vi "Set_Power_Ref(SA).vi"(0 "Spectrum Analyzer":refnum<visa-resource-name>="TCPIP0::K-N90X0A-00005.local::inst0::INSTR", 1 "P_REF":dbl=41.5, 3 "SG_Offset":dbl=26.9, 5 "SigGen1":refnum<visa-resource-name>="GPIB0::18::INSTR", 9 "RF Freq (MHz)":dbl=1840.0, 11 "error in (no error)":errorcluster {"code" format="%.0x"}, 12 "Start Power (dBm)":dbl=15.0, 13 "accuracy +/-":sgl(ring)=0.2 items=["0.1"=0.1, "0.2"=0.2, "0.3"=0.3, "0.4"=0.4, "0.5"=0.5, "1"=1, "2"=2], 14 "Pin MAX":dbl=25.0) -> (4 "Pin (RF1) str":string="51.03", 6 "Pin (RF)":dbl=51.03, 10 "Elasped time(s)":dbl=8.86637079998036, 15 "error out":errorcluster {"code" format="%.0x"})   [LabVIEW 2018]
panel:
  out "SG_Delay(s)":sgl=2.0
  out "x+y":dbl
  in  "Set to Cont Sweep at End":bool
  in  "SA Timeout":u32=3000
  out "End Time":dbl=154195.45798069998 format="%_19f"
  out "Start Time":dbl=154186.5916099 format="%_19f"
  out "ONE_SHOT_Pin":dbl=24.728961346
  out "One Shot >?":bool=TRUE
  out "ONE_SHOT_Pout":dbl=41.992924491
  out "In Range?":bool=TRUE
  out "INIT_DELTA":dbl=9.728961345999998
  out "INIT_GAIN":dbl=16.771038654
  out "INIT_Pout":dbl=31.771038654
  out "P_REF_H":dbl=41.70000000298023
  out "P_REF_L":dbl=41.399999998509884
  out "Power (dBm)":dbl=41.430916708
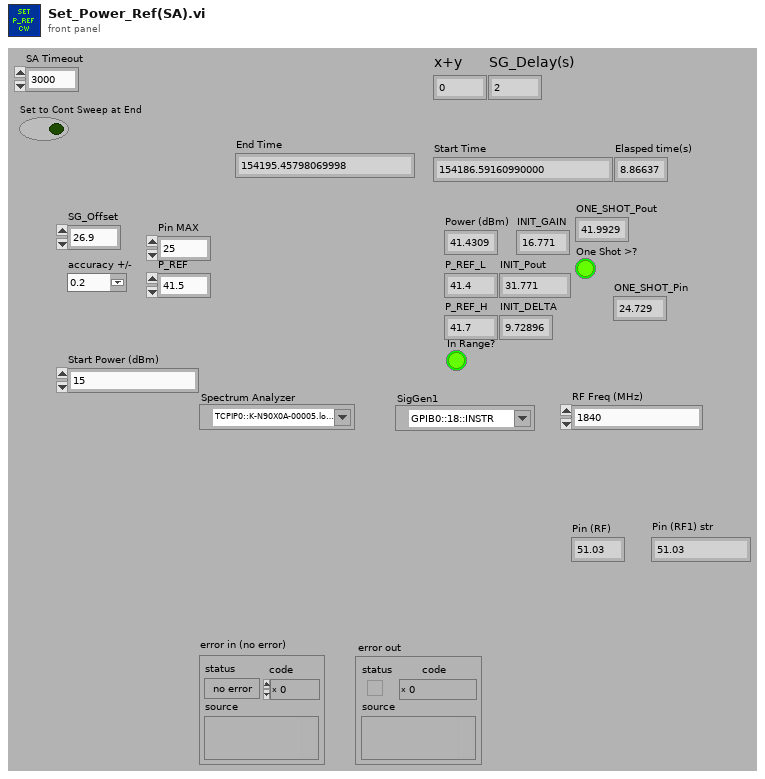
[diagram p1: front panel]
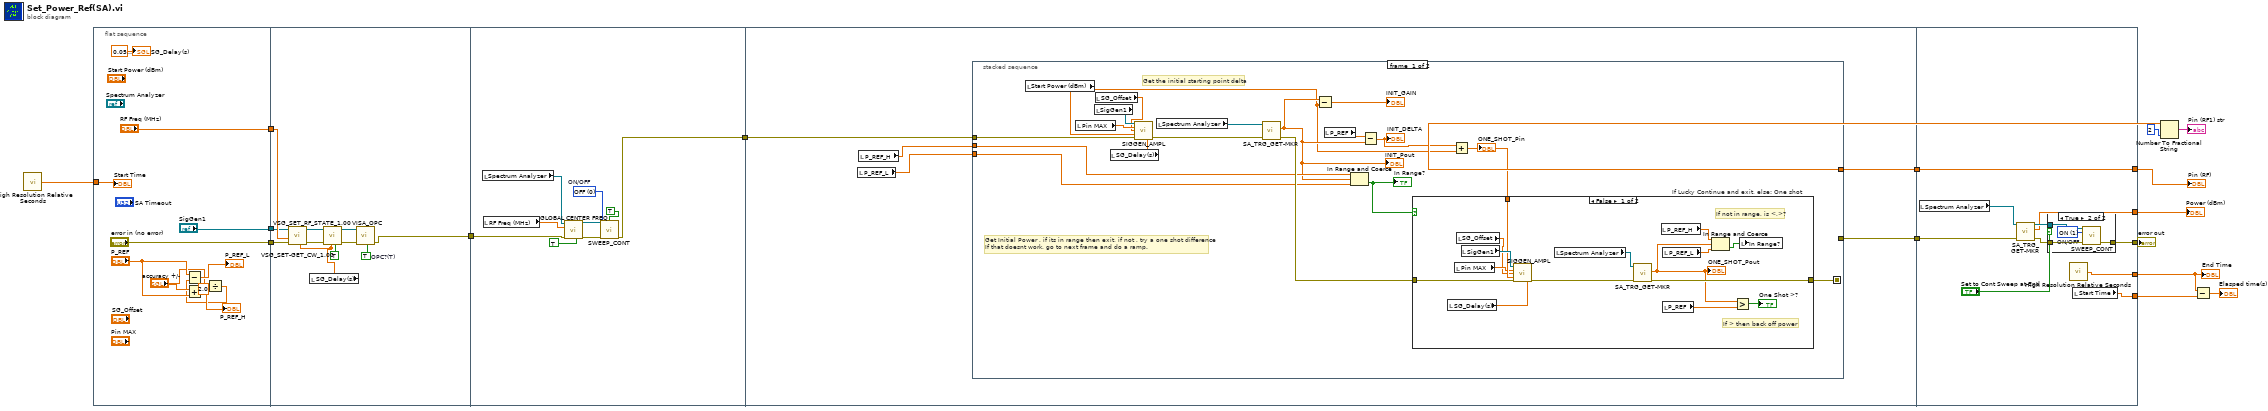
[diagram p0: block diagram]
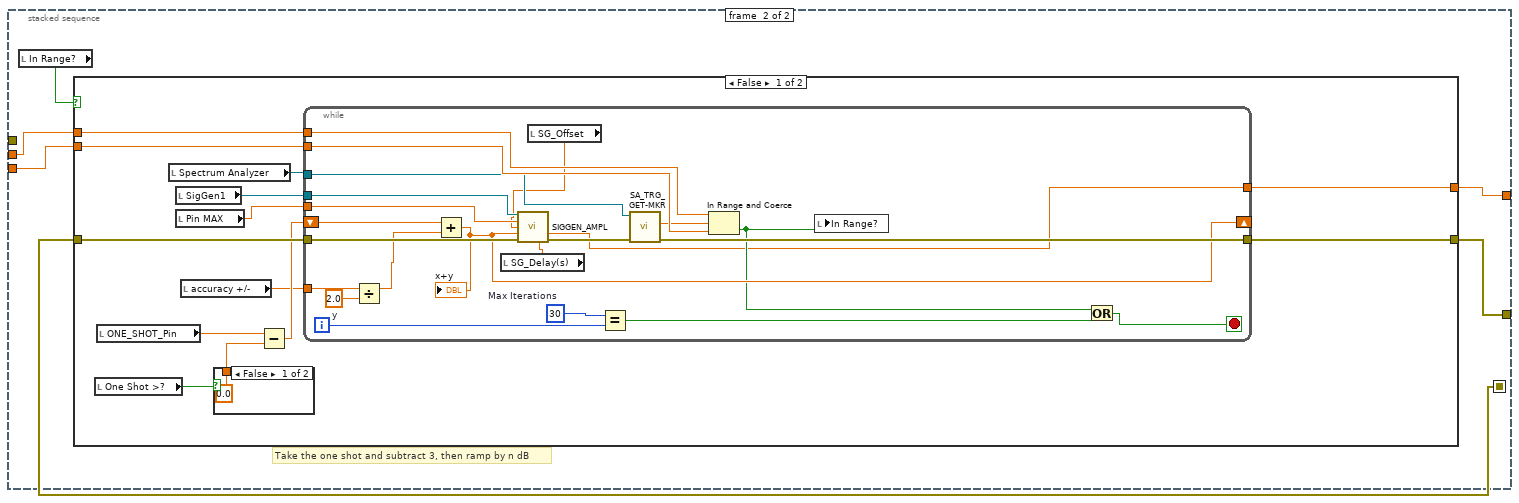
[diagram p3: hidden frame]
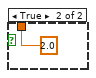
[diagram p4: hidden frame]
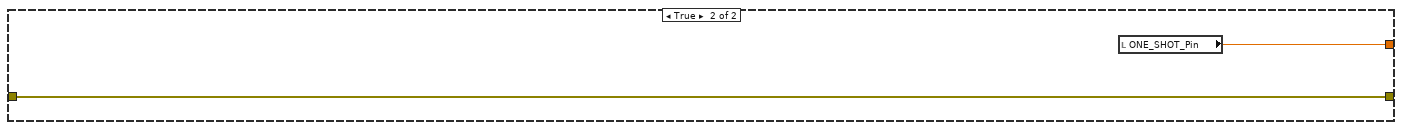
[diagram p5: hidden frame]
diagram:
  n1 = call <vilib>:"High Resolution Relative Seconds.vi"() -> ("relative seconds"=w2:dbl)
  n2 = flat-sequence {
    tunnel: ["error in (no error)"] -> w16
    tunnel: ["RF Freq (MHz)"] -> w15
    tunnel: ["SigGen1"] -> w9
    tunnel: w2 -> [w21]
    tunnel: w16 -> [w37]
    tunnel: w15 -> [w38]
    tunnel: w9 -> [w36]
    tunnel: [w30] -> w8
    tunnel: w8 -> [w44]
    tunnel: [w40] -> w7
    tunnel: [w48] -> w14
    tunnel: [w49] -> w13
    tunnel: w7 -> [w50]
    tunnel: w14 -> [w140]
    tunnel: w13 -> [w141]
    tunnel: [w141] -> w12
    tunnel: [w137] -> w6
    tunnel: [w136] -> w5
    tunnel: [w134] -> w4
    tunnel: [w133] -> w1
    frame #0 {
      n3 = Add(x="accuracy +/-", y="P_REF") -> (x+y=→"P_REF_H":dbl)
      n4 = Divide(x="accuracy +/-", y=sgl 2.0) -> (x/y=w19:sgl)
      n5 = Subtract(x="P_REF", y=w19) -> (x-y=→"P_REF_L":dbl)
      "Start Time" <- w21
      "SG_Delay(s)" <- sgl 0.05 ("y")
    }
    frame #1 {
      w29 = TRUE  # OPC?(T)
      n6 = local read "SG_Delay(s)"() -> (w28:sgl)
      n7 = call "VSG_SET-GET_CW_1.00.vi"("Set Delay after (ms)"=w28, "error in"=w37, "Set Freq (MHz) num"=w38, "Session In"=w36) -> ("error out"=w35:errorcluster, "Session Out"=w34:refnum<visa-resource-name>)  [unwired: 4 in, 2 out]
      n8 = call "VSG_SET_RF_STATE_1.00.vi"("RF ON/OFF (OFF)"=TRUE, "Delay Time (ms)"=w28, "error in"=w35, "Session In"=w34) -> ("error out"=w32:errorcluster, "Session Out"=w31:refnum<visa-resource-name>)  [unwired: 5 in, 1 out]
      n9 = call "VISA_OPC.vi"("OPC(T)"=w29, "error in"=w32, "Session In"=w31) -> ("error out"=w30:errorcluster)  [unwired: 6 in, 2 out]
    }
    frame #2 {
      w39 = u16 0 items=["OFF", "ON"]  # ON/OFF
      n10 = local read "Spectrum Analyzer"() -> (w46:refnum<visa-resource-name>)
      n11 = local read "RF Freq (MHz)"() -> (w47:dbl)
      n12 = call "GLOBAL CENTER FREQ.vi"("Send OPC? (T)"=TRUE, "error in"=w44, "SET CF ()"=w47, "Session In"=w46) -> ("error out"=w43:errorcluster, "Session Out"=w42:refnum<visa-resource-name>)  [unwired: 5 in, 1 out]
      n13 = call "SWEEP_CONT.vi"("Session In"=w42, "OPC?"=TRUE ("OPC?(T)"), "ON/OFF"=w39, "error in"=w43) -> ("error out"=w40:errorcluster)  [unwired: 9 in, 2 out]
    }
    frame #3 {
      n14 = local read "P_REF_L"() -> (w51:dbl)
      n15 = local read "P_REF_H"() -> (w52:dbl)
      n16 = stacked-sequence {
        seq-local: [w62 _] -> [_ w90]
        tunnel: w52 -> [w61 w92]
        tunnel: w51 -> [w60 w91]
        tunnel: w50 -> [w70 _]
        tunnel: [_ w89] -> w49
        tunnel: [_ w87] -> w48
        frame #0 {
          # "Get Initial Power , if its in range then exit, if not , try a one shot difference\nIf that doesnt work, go to next frame and do a ramp."
          # "Get the initial starting point delta"
          n17 = local read "Start Power (dBm)"() -> (w54:dbl)
          n18 = local read "Pin MAX"() -> (w56:dbl)
          n19 = local read "SigGen1"() -> (w68:refnum<visa-resource-name>)
          n20 = local read "SG_Offset"() -> (w53:dbl)
          n21 = local read "SG_Delay(s)"() -> (w67:sgl)
          n22 = call "SIGGEN_AMPL.vi"("Session In"=w68, "Max Power"=w56, "OFFS_IN"=w53, "Set Power (num)"=w54, "error in"=w70, "delay after set (ms)"=w67) -> ("error out"=w69:errorcluster)  [unwired: 6 in, 3 out]
          n23 = local read "Spectrum Analyzer"() -> (w66:refnum<visa-resource-name>)
          n24 = call "SA_TRG_GET-MKR.vi"("error in"=w69, "Session In"=w66) -> ("error out"=w63:errorcluster, "Ampl"=w55:dbl)  [unwired: 7 in, 1 out]
          "INIT_Pout" <- w55
          n25 = Subtract(x=w55, y=w54) -> (x-y=→"INIT_GAIN":dbl)
          n26 = local read "P_REF"() -> (w64:dbl)
          n27 = In Range and Coerce(upper limit=w61, x=w55, lower limit=w60) -> (In Range?=w59:bool)  [unwired: 1 out]
          "In Range?" <- w59
          n28 = Subtract(x=w64, y=w55) -> (x-y=w58:dbl)
          "INIT_DELTA" <- w58
          n29 = Add(x=w58, y=w54) -> (x+y=w57:dbl)
          "ONE_SHOT_Pin" <- w57
          n30 = case "If Lucky Continue and exit, else: One shot" shown="False" w59 {
            tunnel: w63 -> [w85 w86]
            tunnel: [w83 w86] -> w62
            tunnel: w57 -> [w80 _]
            frame False {
              # "If > then back off power"
              # "If not in range, is <,>?"
              n31 = local read "SG_Delay(s)"() -> (w71:sgl)
              n32 = local read "Pin MAX"() -> (w73:dbl)
              n33 = local read "SG_Offset"() -> (w72:dbl)
              n34 = local read "SigGen1"() -> (w82:refnum<visa-resource-name>)
              n35 = call "SIGGEN_AMPL.vi"("Session In"=w82, "Max Power"=w73, "OFFS_IN"=w72, "Set Power (num)"=w80, "error in"=w85, "delay after set (ms)"=w71) -> ("error out"=w84:errorcluster)  [unwired: 6 in, 3 out]
              n36 = local read "Spectrum Analyzer"() -> (w81:refnum<visa-resource-name>)
              n37 = call "SA_TRG_GET-MKR.vi"("error in"=w84, "Session In"=w81) -> ("error out"=w83:errorcluster, "Ampl"=w76:dbl)  [unwired: 7 in, 1 out]
              "ONE_SHOT_Pout" <- w76
              n38 = local read "P_REF_H"() -> (w79:dbl)
              n39 = local read "P_REF"() -> (w75:dbl)
              n40 = local read "P_REF_L"() -> (w78:dbl)
              n41 = In Range and Coerce(upper limit=w79, x=w76, lower limit=w78) -> (In Range?=w77:bool)  [unwired: 1 out]
              n42 = Greater?(x=w76, y=w75) -> (0:→"One Shot >?":bool)
              n43 = local write "In Range?"(w77) -> ()
            }
            frame True {
            }
          }
        }
        frame #1 {
          # "Take the one shot and subtract 3, then ramp by n dB"
          n44 = local read "In Range?"() -> (w88:bool)
          n45 = case shown="False" w88 {
            tunnel: w92 -> [w105 _]
            tunnel: w91 -> [w96 _]
            tunnel: w90 -> [w104 w131]
            tunnel: [w94 w130] -> w89
            tunnel: [w103 w131] -> w87
            frame False {
              n46 = local read "One Shot >?"() -> (w97:bool)
              n47 = local read "ONE_SHOT_Pin"() -> (w100:dbl)
              n48 = local read "Spectrum Analyzer"() -> (w102:refnum<visa-resource-name>)
              n49 = local read "SigGen1"() -> (w101:refnum<visa-resource-name>)
              n50 = local read "Pin MAX"() -> (w95:dbl)
              n51 = local read "accuracy +/-"() -> (w93:sgl)
              n52 = case shown="False" w97 {
                tunnel: [0.0 ("y") 2.0 ("y")] -> w99
                frame False {
                }
                frame True {
                }
              }
              n53 = Subtract(x=w100, y=w99) -> (x-y=w98:dbl)
              n54 = while {
                tunnel: w102 -> [w123]
                tunnel: [w125] -> w103
                tunnel: w104 -> [w129]
                tunnel: w105 -> [w128]
                tunnel: w96 -> [w127]
                tunnel: w101 -> [w122]
                shift-right: [w116] -> _
                shift-left: w98 -> [w121]
                tunnel: w95 -> [w115]
                tunnel: w93 -> [w114]
                tunnel: [w112] -> w94
                i -> [w119]
                stop <- w120 stop-if-true
                w109 = sgl 2.0  # y
                w118 = 30  # Max Iterations
                n55 = Divide(x=w114, y=w109) -> (x/y=w110:sgl)
                n56 = Add(x=w121, y=w110) -> (x+y=w116:dbl)
                "x+y" <- w116
                n57 = local read "SG_Delay(s)"() -> (w108:sgl)
                n58 = local read "SG_Offset"() -> (w111:dbl)
                n59 = call "SIGGEN_AMPL.vi"("Session In"=w122, "Max Power"=w115, "OFFS_IN"=w111, "Set Power (num)"=w116, "error in"=w129, "delay after set (ms)"=w108) -> ("Get Power"=w112:dbl, "error out"=w124:errorcluster)  [unwired: 6 in, 2 out]
                n60 = Equal?(x=w118, y=w119) -> (x = y?=w117:bool)
                n61 = call "SA_TRG_GET-MKR.vi"("error in"=w124, "Session In"=w123) -> ("error out"=w125:errorcluster, "Ampl"=w126:dbl)  [unwired: 7 in, 1 out]
                n62 = In Range and Coerce(upper limit=w128, x=w126, lower limit=w127) -> (In Range?=w113:bool)  [unwired: 1 out]
                n63 = local write "In Range?"(w113) -> ()
                n64 = Or(x=w113, y=w117) -> (x .or. y?=w120:bool)
              }
            }
            frame True {
              n65 = local read "ONE_SHOT_Pin"() -> (w130:dbl)
            }
          }
        }
      }
    }
    frame #4 {
      n66 = local read "Spectrum Analyzer"() -> (w135:refnum<visa-resource-name>)
      n67 = call "SA_TRG_GET-MKR.vi"("error in"=w140, "Session In"=w135) -> ("error out"=w139:errorcluster, "Ampl"=w136:dbl, "Session Out"=w138:refnum<visa-resource-name>)  [unwired: 7 in]
      n68 = case shown="True" "Set to Cont Sweep at End" {
        tunnel: w139 -> [w142 w146]
        tunnel: w138 -> [_ w145]
        tunnel: [w142 w144] -> w137
        frame False {
        }
        frame True {
          w143 = u16 1 items=["OFF", "ON"]  # ON/OFF
          n69 = call "SWEEP_CONT.vi"("Session In"=w145, "ON/OFF"=w143, "error in"=w146) -> ("error out"=w144:errorcluster)  [unwired: 10 in, 2 out]
        }
      }
      n70 = call <vilib>:"High Resolution Relative Seconds.vi"() -> ("relative seconds"=w134:dbl)
      n71 = local read "Start Time"() -> (w133:dbl)
    }
  }
  n72 = Number To Fractional String(number=w12, precision (6)=i16 2) -> (F-format string=→"Pin (RF1) str":string)  [unwired: 2 in]
  n73 = Subtract(x=w4, y=w1) -> (x-y=→"Elasped time(s)":dbl)
  "error out" <- w6
  "Pin (RF)" <- w12
  "Power (dBm)" <- w5
  "End Time" <- w4
